vi "Clean.vi"(0 "VIP in":refnum<class "VIP.lvclass">) -> (4 "VIP out":refnum<class "VIP.lvclass">)   [LabVIEW 2017, in "CL_G3_VIComponentBuilder.lvlib" / "VIP.lvclass"]
doc: "Unregisters and deletes all vi packages found in the export directory. Also deletes the vipb from the export directory"
uses:
  VIP.lvclass
  C:/builds/Component BuilderBT/SrcDist/Exports/Exports/Export.lvclass
  Exports/Export.lvclass/Export.ctl
  Exports/Accessors/Read Component Export Dir.vi
  Exports/Accessors/Read unique Name.vi
  Exports/Accessors/Write Export Operation Errors.vi
  Exports/Accessors/Read Export Operation Errors.vi
  Exports/Export.lvclass
  CL_G3_VIComponentBuilder.lvlib
  VIPM Utilities/CL_G3_VIPMUtilities.lvlib
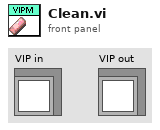
[diagram p1: front panel]
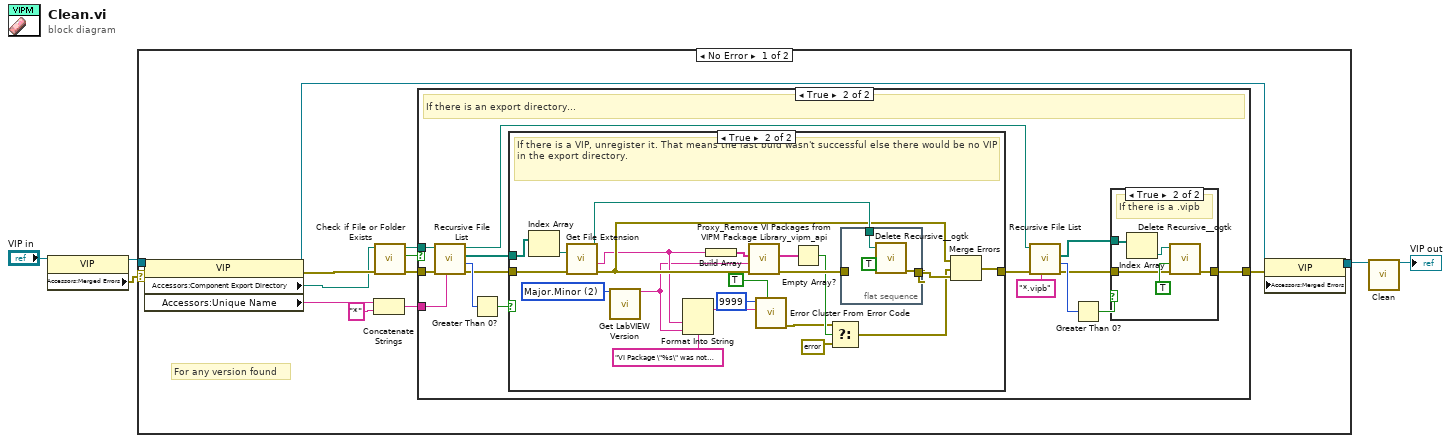
[diagram p0: block diagram]
diagram:
  n1 = property class="VIP"(reference="VIP in") -> (reference out=w2:refnum<class "VIP.lvclass">, "Accessors:Merged Errors"=w1:errorcluster)  [unwired: 1 in, 1 out]
  n2 = case shown="No Error" w1 {
    tunnel: w2 -> [w12 w65]
    tunnel: [w8 w65] -> w5
    frame No Error {
      # "For any version found"
      n3 = property class="VIP"(reference=w12) -> (reference out=w9:refnum<class "VIP.lvclass">, error out=w14:errorcluster, "Accessors:Component Export Directory"=w6:path, "Accessors:Unique Name"=w11:string)  [unwired: 1 in]
      n4 = Concatenate Strings(w11, "*" ("string")) -> (w10:string)
      n5 = call <vilib>:"Check if File or Folder Exists.vi"("error in (no error)"=w14, "path"=w6) -> ("error out"=w13:errorcluster, "file or folder exists?"=w15:bool, "dup path"=w16:path)  [unwired: 7 in]
      n6 = case shown="True" w15 {
        tunnel: w10 -> [_ w33]
        tunnel: w16 -> [_ w29]
        tunnel: w13 -> [w18 w28]
        tunnel: [w18 w20] -> w7
        frame False {
        }
        frame True {
          # "If there is an export directory..."
          n7 = call <vilib>:"Recursive File List.vi"("pattern"=w33, "error in (no error)"=w28, "Folder Path"=w29) -> ("error out"=w27:errorcluster, "Number of Files"=w32:i32, "All Files in Dir"=w31:path[], "dup Folder Path"=w26:path)  [unwired: 4 in, 1 out]
          n8 = Greater Than 0?(x=w32) -> (x > 0?=w30:bool)
          n9 = case shown="True" w30 {
            tunnel: w31 -> [_ w60]
            tunnel: w27 -> [w40 w59]
            tunnel: [w40 w55] -> w22
            frame False {
            }
            frame True {
              w53 = u16 2 items=["Major"=1, "Major.Minor"=2, "Major.Minor.Fix"=3] ("Type Of LabVIEW Version Descriptor")
              # "If there is a VIP, unregister it. That means the last buld wasn't successful else there would be no VIP in the export directory."
              n10 = Index Array(array=w60) -> (element=w58:path)  [unwired: 1 in]
              n11 = call <vilib>:"Get File Extension.vi"("error in (no error)"=w59, "file"=w58) -> ("error out"=w51:errorcluster, "filename without extension"=w46:string, "dup file"=w57:path)  [unwired: 5 in, 2 out]
              n12 = call "Get LabVIEW Version.vi"("Type Of LabVIEW Version Descriptor"=w53) -> ("LabVIEW Version"=w45:string)  [unwired: 13 in, 1 out]
              n13 = Format Into String(format string="VI Package \"%s\" was not removed for LabVIEW Version %s", w46, w45) -> (resulting string=w44:string)  [unwired: 2 in, 1 out]
              n14 = Build Array(w46) -> (w61:string[])
              n15 = call "Proxy_Remove VI Packages from VIPM Package Library_vipm_api.vi"("error in (no error)"=w51, "LabVIEW Version"=w45, "Package Names to Remove"=w61) -> ("error out"=w54:errorcluster, "Packages Removed"=w52:string[])  [unwired: 7 in]
              n16 = call <vilib>:"Error Cluster From Error Code.vi"("show call chain? (False)"=TRUE, "error message (\"\")"=w44, "error code (0)"=9999) -> ("error out"=w43:errorcluster)  [unwired: 6 in]
              n17 = Empty Array?(array=w52) -> (empty?=w50:bool)
              n18 = Select(t=w43, s=w50, f=errorcluster {"status"=FALSE, "code"=0, "source"=""} ("error out")) -> (s? t:f=w48:errorcluster)
              n19 = flat-sequence {
                tunnel: w57 -> [w63]
                tunnel: [w62] -> w56
                tunnel: w54 -> [_]
                frame #0 {
                  n20 = call <userlib>:"Delete Recursive__ogtk.vi"("Ignore Read-Only? (FALSE)"=TRUE, "Path"=w63) -> ("error out"=w62:errorcluster)  [unwired: 8 in, 1 out]
                }
              }
              n21 = Merge Errors(w51, w48, w56) -> (w55:errorcluster)
            }
          }
          n22 = call <vilib>:"Recursive File List.vi"("pattern"="*.vipb", "error in (no error)"=w22, "Folder Path"=w26) -> ("error out"=w21:errorcluster, "Number of Files"=w25:i32, "All Files in Dir"=w23:path[])  [unwired: 4 in, 2 out]
          n23 = Greater Than 0?(x=w25) -> (x > 0?=w24:bool)
          n24 = case shown="True" w24 {
            tunnel: w23 -> [_ w39]
            tunnel: w21 -> [w34 w36]
            tunnel: [w34 w35] -> w20
            frame False {
            }
            frame True {
              # "If there is a .vipb"
              n25 = Index Array(array=w39) -> (element=w38:path)  [unwired: 1 in]
              n26 = call <userlib>:"Delete Recursive__ogtk.vi"("error in (no error)"=w36, "Ignore Read-Only? (FALSE)"=TRUE, "Path"=w38) -> ("error out"=w35:errorcluster)  [unwired: 7 in, 1 out]
            }
          }
        }
      }
      n27 = property class="VIP"(reference=w9, "Accessors:Merged Errors"=w7) -> (reference out=w8:refnum<class "VIP.lvclass">)  [unwired: 1 in, 1 out]
    }
    frame Error {
    }
  }
  n28 = call-parent "Clean.vi"("Export in"=w5) -> ("Export out"=→"VIP out":refnum<class "VIP.lvclass">)  [unwired: 14 in]
